vi "RubikStartState.vi"() -> (0 "error out":errorcluster)   [LabVIEW 2017, in "RubikLibraryRT.lvlib"]
uses:
  RubikLibraryRT.lvlib
  ServoEnumControl.ctl
  ServoAbsAngleControl.ctl
  <vilib>/ErrorRing/Error Ring.xnode
  RubikLibrary.lvlib
panel:
  in  "List of Servo Angles":T1[](array[typedef])
  in  "Gripper closed":bool=TRUE
  in  "List of Servos":T2[](array[typedef])=[enum."Left Servo", enum."Front Servo", enum."Right Servo"]
  # "Rubic Start"
  # "Rubik Cube Start Configuration\n\nPosition of Grippers:  Closed\nPosition of Servos: 0°"
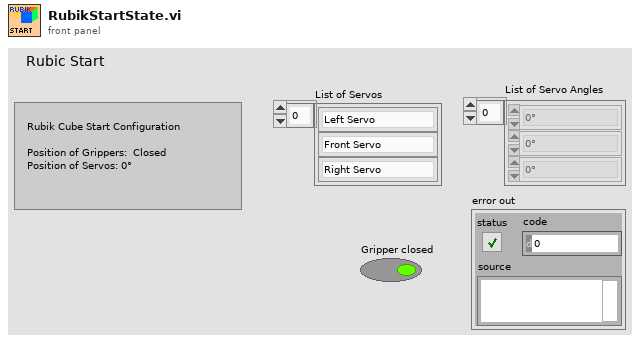
[diagram p1: front panel]
types:
  T1 = typedef "RubikLibrary.lvlib/ServoAbsAngleControl.ctl" = enum16{"+90°", "0°", "-90°"}
  T2 = typedef "RubikLibrary.lvlib/ServoEnumControl.ctl" = enum16{"Left Servo", "Front Servo", "Right Servo"}
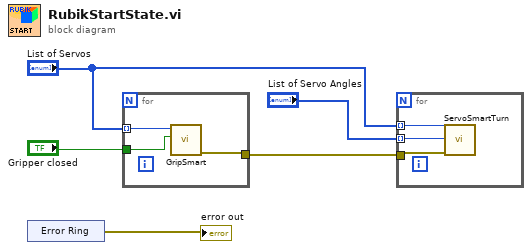
[diagram p0: block diagram]
diagram:
  n1 = xnode "Error Ring"() -> ("error out"=→"error out":errorcluster)
  n2 = for {
    tunnel: "List of Servos" -> [w8] mode=indexing
    tunnel: "Gripper closed" -> [w7]
    tunnel: [w6] -> w3
    n3 = call "GripSmart.vi"("Grip closed (in)"=w7, "Servo"=w8) -> ("error out"=w6:errorcluster)  [unwired: 8 in, 1 out]
  }
  n4 = for {
    tunnel: "List of Servos" -> [w11] mode=indexing
    tunnel: w3 -> [w10]
    tunnel: "List of Servo Angles" -> [w9] mode=indexing
    n5 = call "ServoSmartTurn.vi"("error in"=w10, "Turn to (in)"=w9, "Servo"=w11) -> ()  [unwired: 7 in, 2 out]
  }
